vi "Cleanup.vi"(8 "error in (no error)":errorcluster, 11 "Builder in":refnum<class "Builder.lvclass">) -> (0 "error out":errorcluster)   [LabVIEW 2020, in "Builder Tools.lvlib" / "Builder.lvclass"]
uses:
  Builder.lvclass
  Builder.lvclass/Builder.ctl
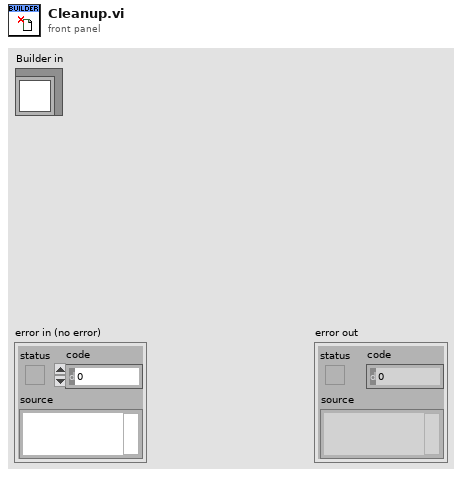
[diagram p1: front panel]
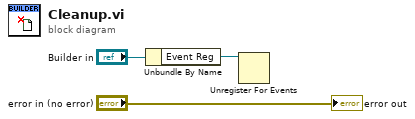
[diagram p0: block diagram]
diagram:
  n1 = Unbundle By Name("Builder in") -> ("Event Reg"=w1:refnum<event-registration>)
  n2 = Unregister For Events(event registration refnum=w1) -> ()  [unwired: 1 in, 1 out]
  "error out" <- "error in (no error)"
